vi "Stop Core.vi"(10 "final error code":i32, 11 "VisionUI in":refnum<class "VisionUI.lvclass">) -> (3 "VisionUI out":refnum<class "VisionUI.lvclass">)   [LabVIEW 2021, in "VisionUI.lvlib" / "VisionUI.lvclass"]
doc: "(<B>Filename</B>: Actor Framework.lvlib:Actor.lvclass:Stop Core.vi)\n\nDefines what the actor does before it stops. Use the <B>final error code</B> input to determine whether the actor shut down in response to an error.\n\nBy default, this method passes the Stop message along to all auto-stop nested actors. A descendant class may override this method to define additional behavior, such as shutting down any processes the actor initiated in its override of the Actor Core method."
uses:
  VisionUI.lvclass
  VisionUI.lvclass/VisionUI.ctl
  Vision/Vision/Vision.lvclass
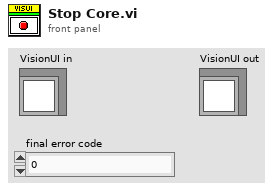
[diagram p1: front panel]
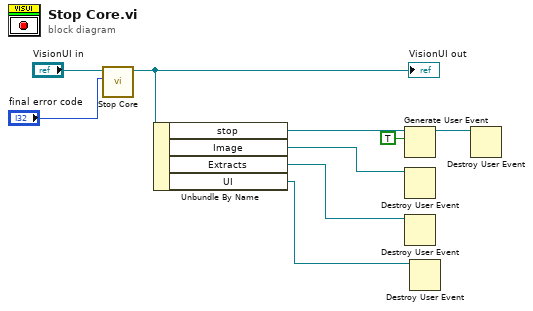
[diagram p0: block diagram]
diagram:
  n1 = call-parent "Stop Core.vi"("final error code"="final error code", "Vision in"="VisionUI in") -> ("Vision out"=w7:refnum<class "VisionUI.lvclass">)  [unwired: 9 in]
  "VisionUI out" <- w7
  n2 = Unbundle By Name(w7) -> ("stop"=w6:refnum<user-event>, "Image"=w3:refnum<user-event>, "Extracts"=w2:refnum<user-event>, "UI"=w1:refnum<user-event>)
  n3 = Generate User Event(user event=w6, event data cluster=TRUE ("event data")) -> (user event out=w4:refnum<user-event>)  [unwired: 2 in, 1 out]
  n4 = Destroy User Event(user event=w3) -> ()  [unwired: 1 in, 1 out]
  n5 = Destroy User Event(user event=w2) -> ()  [unwired: 1 in, 1 out]
  n6 = Destroy User Event(user event=w1) -> ()  [unwired: 1 in, 1 out]
  n7 = Destroy User Event(user event=w4) -> ()  [unwired: 1 in, 1 out]
